vi "CountingFPGA.vi"() -> ()   [LabVIEW 2016]
uses:
  <vilib>/rvi/Emulation/niFpgaGetClockAttributes.vi
  <vilib>/rvi/Emulation/niFpgaSctlEmulationGetInTimedLoop.vi
  <vilib>/rvi/Emulation/niFpgaEmulationReportErrorSimple.vi
  <vilib>/rvi/Emulation/niFpgaProcessEmulError.vi
  <vilib>/rvi/eio/common/nirviEmuTemplateMethod_errors.vi
  <vilib>/rvi/Emulation/niFpgaCriticalErrorInLSC.vi
  <vilib>/eio/EIONode/EIONode.xnode
panel:
  out "vHR":sgl
  out "vHL":sgl
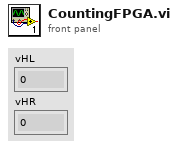
[diagram p1: front panel]
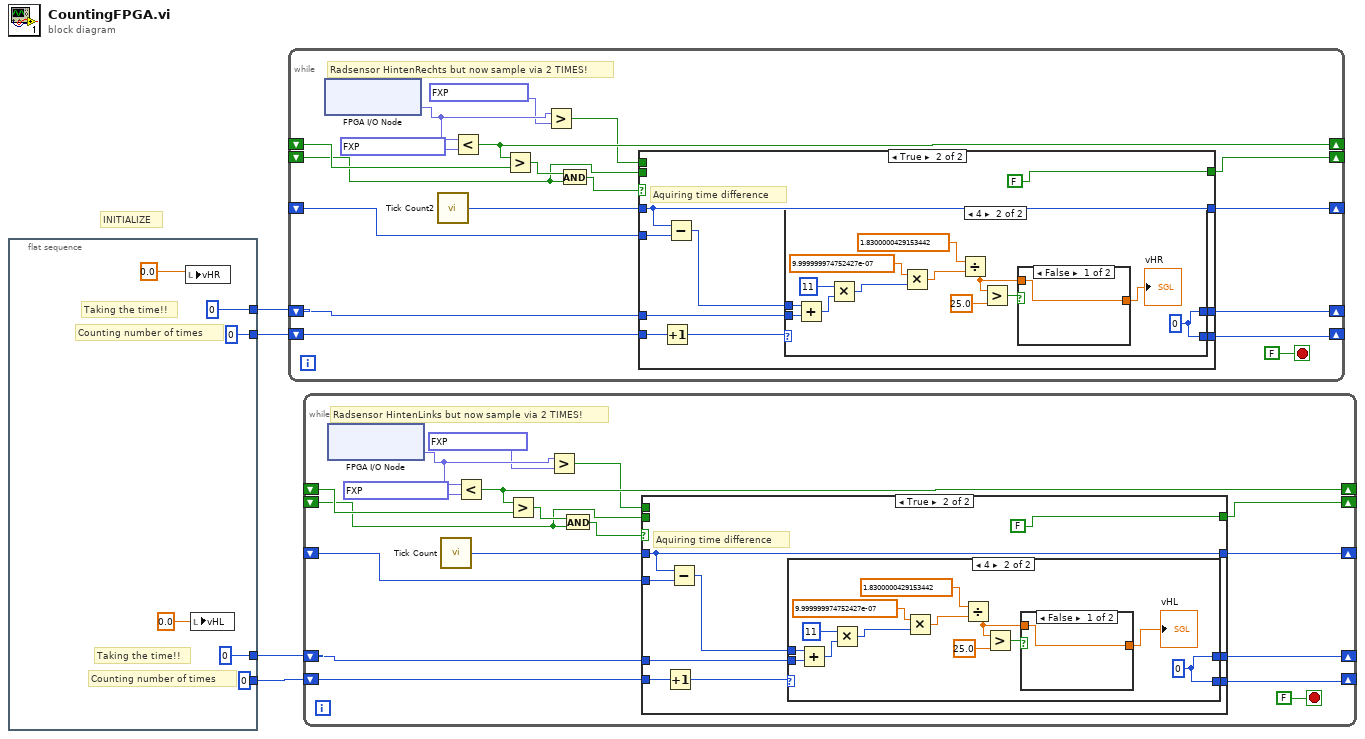
[diagram p0: block diagram]
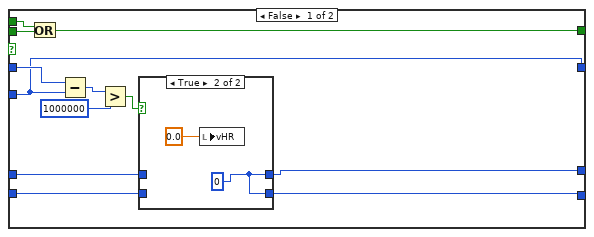
[diagram p2: hidden frame]
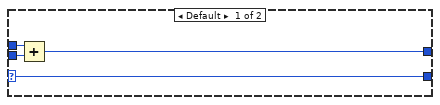
[diagram p4: hidden frame]
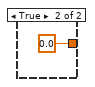
[diagram p5: hidden frame]
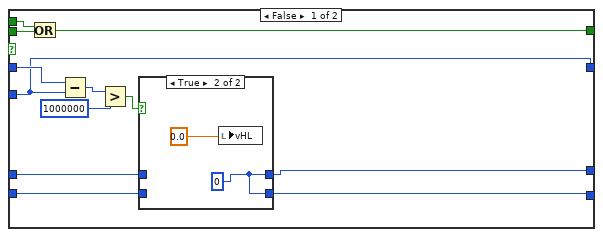
[diagram p6: hidden frame]
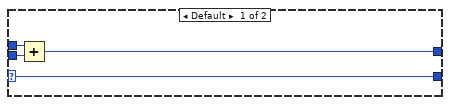
[diagram p8: hidden frame]
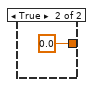
[diagram p9: hidden frame]
diagram:
  # "INITIALIZE"
  n1 = flat-sequence {
    tunnel: [i16 0] -> w4
    tunnel: [i16 0] -> w3
    tunnel: [i16 0] -> w2
    tunnel: [i16 0] -> w1
    frame #0 {
      # "Taking the time!!"
      # "Counting number of times"
      # "Taking the time!!"
      # "Counting number of times"
      n2 = local write "vHR"(sgl 0.0) -> ()
      n3 = local write "vHL"(sgl 0.0) -> ()
    }
  }
  n4 = while {
    shift-right: [w27] -> _
    shift-left: _ -> [w26]
    shift-right: [w24] -> _
    shift-left: _ -> [w23]
    shift-right: [w22] -> _
    shift-left: w1 -> [w21]
    shift-right: [w20] -> _
    shift-left: w2 -> [w19]
    shift-right: [w14] -> _
    shift-left: _ -> [w15]
    stop <- FALSE stop-if-true
    # "Radsensor HintenRechts but now sample via 2 TIMES!"
    n5 = xnode "FPGA I/O Node"() -> ("Mod2/AI0"=w13:fxp<+,18,3>)  [unwired: 1 in, 1 out]
    n6 = call "Tick Count2"() -> ("Tick Count(uSec)"=w25:u32)
    n7 = Less?(x=w13, y=fxp<+,18,3> 0.024993896484375) -> (x < y?=w27:bool)
    n8 = Greater?(x=w27, y=w26) -> (0:w18:bool)
    n9 = Greater?(x=w13, y=fxp<+,18,3> 0.32501220703125) -> (0:w16:bool)
    n10 = And(x=w18, y=w15) -> (x .and. y?=w17:bool)
    n11 = case shown="True" w17 {
      tunnel: w25 -> [w37 w53]
      tunnel: [w36 w53] -> w24
      tunnel: w23 -> [w36 w52]
      tunnel: w21 -> [w30 w51]
      tunnel: [w29 w49] -> w22
      tunnel: w19 -> [w32 w48]
      tunnel: [w31 w46] -> w20
      tunnel: w16 -> [w40 _]
      tunnel: w15 -> [w39 _]
      tunnel: [w38 FALSE] -> w14
      frame False {
        n12 = Or(x=w40, y=w39) -> (x .or. y?=w38:bool)
        n13 = Subtract(x=w37, y=w36) -> (x-y=w34:u32)
        n14 = Greater?(x=w34, y=u32 1000000) -> (0:w35:bool)
        n15 = case shown="True" w35 {
          tunnel: w32 -> [w42 _]
          tunnel: [w42 w44] -> w31
          tunnel: w30 -> [w41 _]
          tunnel: [w41 w44] -> w29
          frame False {
          }
          frame True {
            w44 = 0
            n16 = local write "vHR"(sgl 0.0) -> ()
          }
        }
      }
      frame True {
        # "Aquiring time difference"
        n17 = Increment(x=w51) -> (x+1=w50:i32)
        n18 = Subtract(x=w53, y=w52) -> (x-y=w47:u32)
        n19 = case shown="4" w50 {
          selector: w50 -> [w57 _]
          tunnel: [w57 w70] -> w49
          tunnel: w48 -> [w56 w69]
          tunnel: w47 -> [w55 w68]
          tunnel: [w54 w70] -> w46
          frame Default {
            n20 = Add(x=w55, y=w56) -> (x+y=w54:u32)
          }
          frame 4 {
            w70 = i16 0
            n21 = Add(x=w68, y=w69) -> (x+y=w67:u32)
            n22 = Multiply(x=u32 11, y=w67) -> (x*y=w64:u32)
            n23 = Multiply(x=sgl 1e-06, y=w64) -> (x*y=w62:sgl)
            n24 = Divide(x=sgl 1.83, y=w62) -> (x/y=w60:sgl)
            n25 = Greater?(x=w60, y=sgl 25.0) -> (0:w59:bool)
            n26 = case shown="False" w59 {
              tunnel: w60 -> [w71 _]
              tunnel: [w71 sgl 0.0] -> w58
              frame False {
              }
              frame True {
              }
            }
            "vHR" <- w58
          }
        }
      }
    }
  }
  n27 = while {
    shift-right: [w89] -> _
    shift-left: _ -> [w88]
    shift-right: [w86] -> _
    shift-left: _ -> [w85]
    shift-right: [w84] -> _
    shift-left: w3 -> [w83]
    shift-right: [w82] -> _
    shift-left: w4 -> [w81]
    shift-right: [w76] -> _
    shift-left: _ -> [w77]
    stop <- FALSE stop-if-true
    # "Radsensor HintenLinks but now sample via 2 TIMES!"
    n28 = xnode "FPGA I/O Node"() -> ("Mod2/AI1"=w75:fxp<+,18,3>)  [unwired: 1 in, 1 out]
    n29 = call "Tick Count"() -> ("Tick Count(uSec)"=w87:u32)
    n30 = Less?(x=w75, y=fxp<+,18,3> 0.024993896484375) -> (x < y?=w89:bool)
    n31 = Greater?(x=w89, y=w88) -> (0:w80:bool)
    n32 = Greater?(x=w75, y=fxp<+,18,3> 0.29998779296875) -> (0:w78:bool)
    n33 = And(x=w80, y=w77) -> (x .and. y?=w79:bool)
    n34 = case shown="True" w79 {
      tunnel: w87 -> [w99 w115]
      tunnel: [w98 w115] -> w86
      tunnel: w85 -> [w98 w114]
      tunnel: w83 -> [w92 w113]
      tunnel: [w91 w111] -> w84
      tunnel: w81 -> [w94 w110]
      tunnel: [w93 w108] -> w82
      tunnel: w78 -> [w102 _]
      tunnel: w77 -> [w101 _]
      tunnel: [w100 FALSE] -> w76
      frame False {
        n35 = Or(x=w102, y=w101) -> (x .or. y?=w100:bool)
        n36 = Subtract(x=w99, y=w98) -> (x-y=w96:u32)
        n37 = Greater?(x=w96, y=u32 1000000) -> (0:w97:bool)
        n38 = case shown="True" w97 {
          tunnel: w94 -> [w104 _]
          tunnel: [w104 w106] -> w93
          tunnel: w92 -> [w103 _]
          tunnel: [w103 w106] -> w91
          frame False {
          }
          frame True {
            w106 = 0
            n39 = local write "vHL"(sgl 0.0) -> ()
          }
        }
      }
      frame True {
        # "Aquiring time difference"
        n40 = Increment(x=w113) -> (x+1=w112:i32)
        n41 = Subtract(x=w115, y=w114) -> (x-y=w109:u32)
        n42 = case shown="4" w112 {
          selector: w112 -> [w119 _]
          tunnel: [w119 w132] -> w111
          tunnel: w110 -> [w118 w131]
          tunnel: w109 -> [w117 w130]
          tunnel: [w116 w132] -> w108
          frame Default {
            n43 = Add(x=w117, y=w118) -> (x+y=w116:u32)
          }
          frame 4 {
            w132 = i16 0
            n44 = Add(x=w130, y=w131) -> (x+y=w129:u32)
            n45 = Multiply(x=u32 11, y=w129) -> (x*y=w126:u32)
            n46 = Multiply(x=sgl 1e-06, y=w126) -> (x*y=w124:sgl)
            n47 = Divide(x=sgl 1.83, y=w124) -> (x/y=w122:sgl)
            n48 = Greater?(x=w122, y=sgl 25.0) -> (0:w121:bool)
            n49 = case shown="False" w121 {
              tunnel: w122 -> [w133 _]
              tunnel: [w133 sgl 0.0] -> w120
              frame False {
              }
              frame True {
              }
            }
            "vHL" <- w120
          }
        }
      }
    }
  }
